vi "Pitch(SubVI).vi"(8 "Numeric":i32, 10 "Target radius":dbl=38.0, 11 "Radius in":dbl) -> (2 "Radius out":cluster{dbl, dbl}(knob)={0.0, 38.0}, 3 "Pitch out":sgl)   [LabVIEW 2014]
uses:
  Global.vi
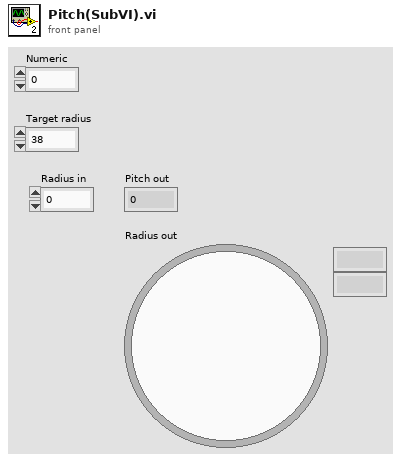
[diagram p1: front panel]
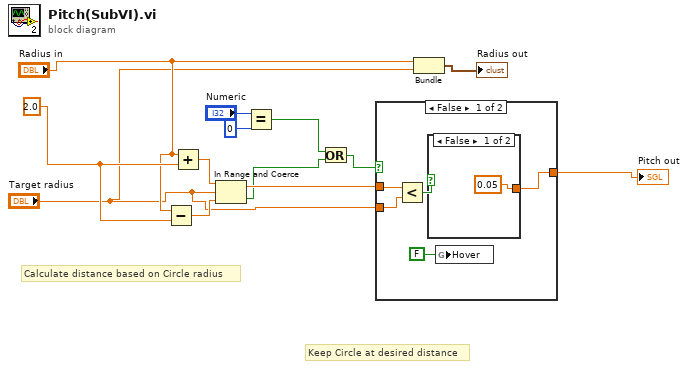
[diagram p0: block diagram]
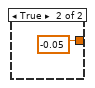
[diagram p2: hidden frame]
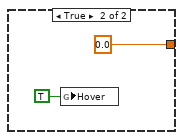
[diagram p3: hidden frame]
diagram:
  w11 = 2.0
  # "Keep Circle at desired distance"
  # "Calculate distance based on Circle radius"
  n1 = Subtract(x="Radius in", y=w11) -> (x-y=w13:dbl)
  n2 = Add(x="Radius in", y=w11) -> (x+y=w12:dbl)
  n3 = In Range and Coerce(upper limit=w12, x="Target radius", lower limit=w13) -> (coerced(x)=w9:dbl, In Range?=w5:bool)
  n4 = Equal?(x="Numeric", y=0) -> (x = y?=w6:bool)
  n5 = Or(x=w6, y=w5) -> (x .or. y?=w4:bool)
  n6 = case shown="False" w4 {
    tunnel: [w18 sgl 0.0 ("Pitch out")] -> w10
    tunnel: w9 -> [w17 _]
    tunnel: "Target radius" -> [w16 _]
    frame False {
      n7 = Less?(x=w17, y=w16) -> (x < y?=w15:bool)
      n8 = case shown="False" w15 {
        tunnel: [0.05 -0.05] -> w18
        frame False {
        }
        frame True {
        }
      }
      n9 = global write "Global.vi" "Hover"(FALSE) -> ()
    }
    frame True {
      n10 = global write "Global.vi" "Hover"(TRUE) -> ()
    }
  }
  "Pitch out" <- w10
  n11 = Bundle("Radius in"="Radius in", "Target radius"="Target radius") -> (→"Radius out":cluster{"Radius in":dbl, "Target radius":dbl})  [unwired: 1 in]
